vi "FGV Daten Abholung uebergeben.vi"(0 "Zustand":string, 1 "aufsteigend":bool, 5 "Anzeige aktualisieren":bool, 7 "Beendet":bool, 9 "Restlaufzeit":sgl, 11 "error in (no error)":errorcluster caption="Fehler (Eingang, kein Fehler)", 13 "Aktion":T1) -> (4 "Zustand":string, 6 "Anzeige aktualisieren":bool, 8 "Beendet":bool, 10 "Restlaufzeit out":sgl, 15 "error out":errorcluster caption="Fehler (Ausgang)")   [LabVIEW 2020, in "Linearisierung v2.lvlib" / "Gasteiler.lvlib"]
uses:
  Gasteiler.lvlib
  Aktion FGV Daten Abholung uebergebenctl.ctl
  Allgemein/allgemeine Sub-VIs.lvlib
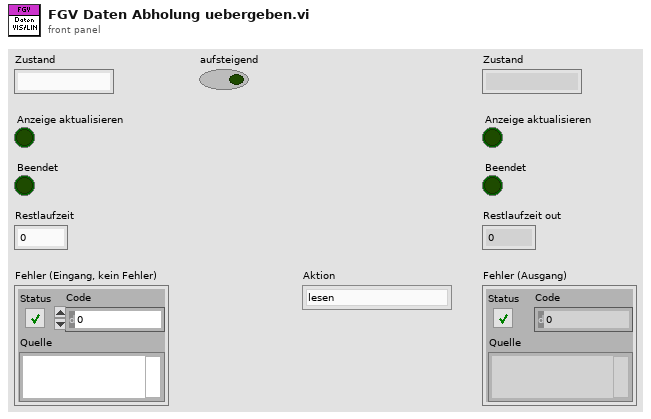
[diagram p1: front panel]
types:
  T1 = typedef "Linearisierung v2.lvlib/Gasteiler.lvlib/Aktion FGV Daten Abholung uebergebenctl.ctl" = enum16{"lesen", "schreiben", "Anzeigebit löschen", "Status hinzufügen"}
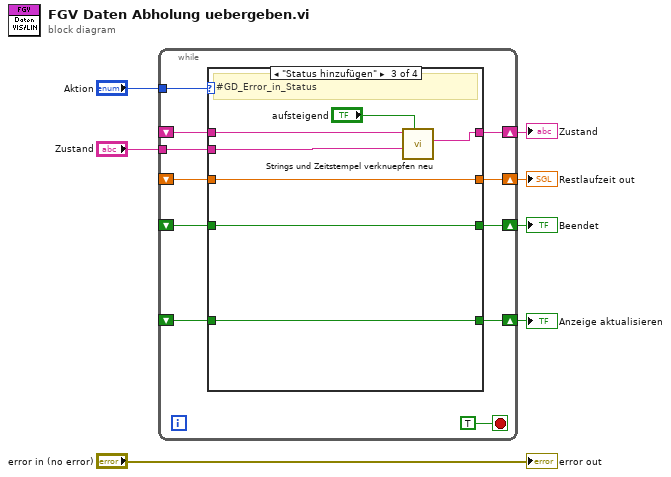
[diagram p0: block diagram]
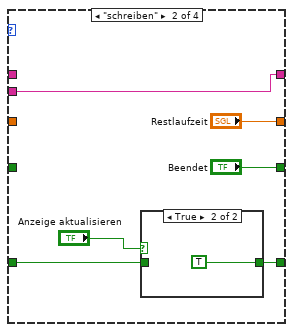
[diagram p3: hidden frame]
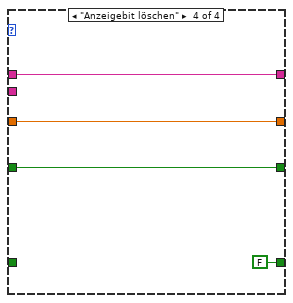
[diagram p5: hidden frame]
diagram:
  n1 = while {
    tunnel: "Aktion" -> [w17]
    shift-right: [w16] -> w6
    shift-left: _ -> [w15]
    shift-right: [w14] -> w5
    shift-left: _ -> [w13]
    shift-right: [w12] -> w4
    shift-left: _ -> [w11]
    shift-right: [w10] -> w3
    shift-left: _ -> [w9]
    tunnel: "Zustand" -> [w8]
    stop <- TRUE stop-if-true
    n2 = case shown="\"Status hinzufügen\"" w17 {
      tunnel: [w22 w23 w34 w41] -> w16
      tunnel: w15 -> [w22 _ w33 w41]
      tunnel: [w21 "Beendet" w37 w40] -> w14
      tunnel: w13 -> [w21 _ w37 w40]
      tunnel: [w20 w26 w35 FALSE ("Beendet")] -> w12
      tunnel: w11 -> [w20 w25 w35 _]
      tunnel: [w19 "Restlaufzeit" w36 w38] -> w10
      tunnel: w9 -> [w19 _ w36 w38]
      tunnel: w8 -> [_ w23 w31 _]
      frame "lesen", Default {
      }
      frame "schreiben" {
        n3 = case shown="True" "Anzeige aktualisieren" {
          tunnel: [w29 TRUE ("Beendet")] -> w26
          tunnel: w25 -> [w29 _]
          frame False {
          }
          frame True {
          }
        }
      }
      frame "Status hinzufügen" {
        # "#GD_Error_in_Status"
        n4 = call "Strings und Zeitstempel verknuepfen neu.vi"("aufsteigend"="aufsteigend", "String 1 hinzufügen"=w31, "Eingangs String"=w33) -> ("Verknüpfter String"=w34:string)  [unwired: 8 in]
      }
      frame "Anzeigebit löschen" {
      }
    }
  }
  "Zustand" <- w6
  "Anzeige aktualisieren" <- w4
  "Beendet" <- w5
  "Restlaufzeit out" <- w3
  "error out" <- "error in (no error)"
